vi "Filter AI Signal - Single.vi"(0 "reference in":refnum<class "AI.lvclass">, 3 "AI Channel Number (Zero Based)":i32, 5 "error in (no error)":errorcluster) -> (14 "reference out":refnum<class "AI.lvclass">, 15 "AI Channel Readings":dbl[](array[numeric]), 16 "AI Channel Sample Average":dbl, 17 "AI Channel Sample Standard Deviation":dbl, 18 "AI Channel Signal is Zero":bool, 19 "error out":errorcluster)   [LabVIEW 2017]
uses:
  AI.lvclass
  <vilib>/Analysis/NI_AALBase.lvlib
  <vilib>/Analysis/3filter.llb/Filter Passband Type.ctl
  <vilib>/Analysis/3filter.llb/Butterworth Filter (DBL).vi
panel:
  out "AI Channel Reading Chart":dbl[](graph)
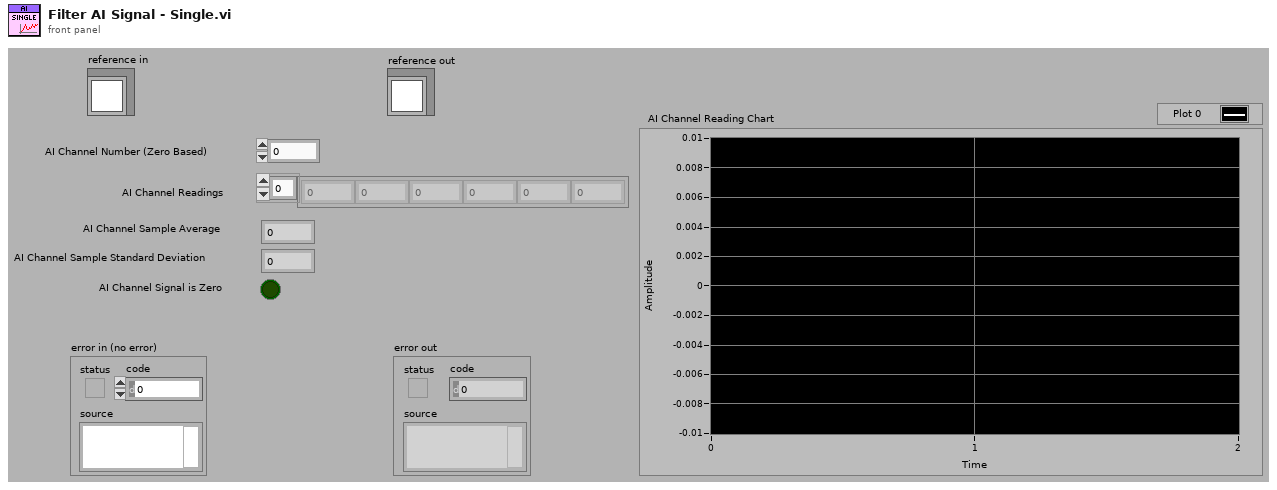
[diagram p1: front panel]
types:
  T1 = typedef "NI_AALBase.lvlib/Filter Passband Type.ctl" = enum32{"Lowpass", "Highpass", "Bandpass", "Bandstop"}
  T2 = typedef "AI.lvclass/ObjectAttributes.ctl" = cluster{"AI Task":refnum<k21>, "AI On/Off Status":bool, "AI Sampling Rate (Samples/Seconds)":u32, "Number of AI Samples Per Channel":i32, "AI Voltage Range":u8, "AI Readings":dbl[][], "Number of AI Modules":i32, "Number of Total AI Channels":i32, "AI Module Names (NI-Max Name)":string[], "Number of Channels Per AI  Module":i32[], "AI VI Reference":refnum<vi>}
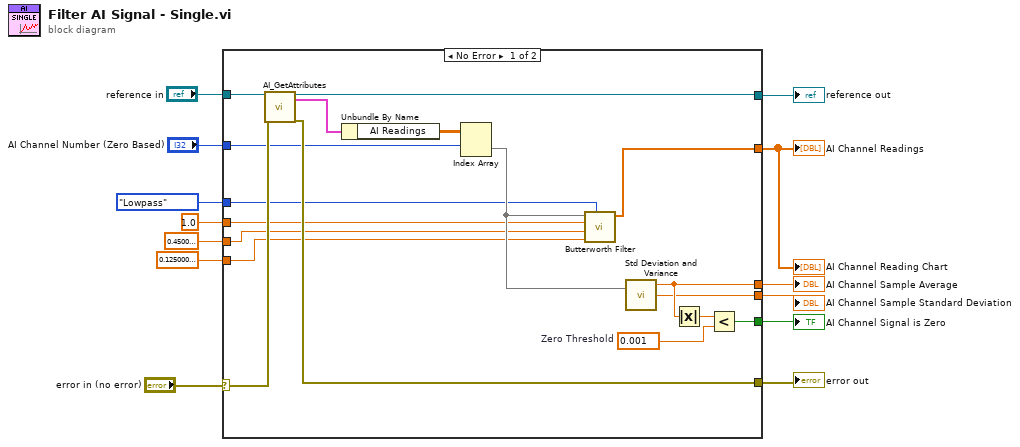
[diagram p0: block diagram]
diagram:
  n1 = case shown="No Error" "error in (no error)" {
    selector: "error in (no error)" -> [w30 w33]
    tunnel: [w28 w33] -> w12
    tunnel: [w29 w32] -> w10
    tunnel: "reference in" -> [w31 w32]
    tunnel: "AI Channel Number (Zero Based)" -> [w27 _]
    tunnel: [w26 _] -> w6
    tunnel: [w25 _] -> w8
    tunnel: [w24 _] -> w7
    tunnel: [w17 _] -> w5
    tunnel: Filter_Passband_Type."Lowpass" ("filter type") -> [w18 _]
    tunnel: 1.0 ("sampling freq: fs") -> [w16 _]
    tunnel: 0.45000000000000007 ("high cutoff freq: fh") -> [w15 _]
    tunnel: 0.12500000000000006 ("low cutoff freq: fl") -> [w14 _]
    frame No Error {
      w22 = 0.001  # Zero Threshold
      n2 = call "AI_GetAttributes.vi"("reference in"=w31, "error in (no error)"=w30) -> ("reference out"=w29:refnum<class "AI.lvclass">, "Data"=w20:T2, "error out"=w28:errorcluster)  [unwired: 14 in, 1 out]
      n3 = Unbundle By Name(w20) -> ("AI Readings"=w23:dbl[][])
      n4 = Index Array(array=w23, index (row)=w27) -> (element=w19:dbl[])  [unwired: 1 in]
      n5 = call-poly <vilib>:"Butterworth Filter.vi"("filter type"=w18, "low cutoff freq: fl"=w14, "high cutoff freq: fh"=w15, "sampling freq: fs"=w16, "X"=w19) -> ("Filtered X"=w17:dbl[])  [unwired: 3 in, 1 out]
      n6 = call <vilib>:"Std Deviation and Variance.vi"("X"=w19) -> ("mean"=w26:dbl, "standard deviation"=w24:dbl)  [unwired: 1 in, 1 out]
      n7 = Absolute Value(x=w26) -> (abs(x)=w21:dbl)
      n8 = Less?(x=w21, y=w22) -> (x < y?=w25:bool)
    }
    frame Error {
    }
  }
  "error out" <- w12
  "reference out" <- w10
  "AI Channel Readings" <- w5
  "AI Channel Signal is Zero" <- w8
  "AI Channel Sample Standard Deviation" <- w7
  "AI Channel Sample Average" <- w6
  "AI Channel Reading Chart" <- w5
